vi "Consolidate Data Type.vi"(11 "Type in":T1) -> (3 "Type out":T1)   [LabVIEW 2020, in "hse-config.lvlib" / "config-base.lvclass"]
doc: "____\nHAMPEL SOFTWARE ENGINEERING v3.8.0 (2023-12-18 14:41)"
uses:
  config-base.lvclass
  <vilib>/Utility/Data Type/Type Definitions/Data Type.ctl
  config-base.lvclass/config-base.ctl
  <vilib>/Utility/Data Type/NI_Data Type.lvlib
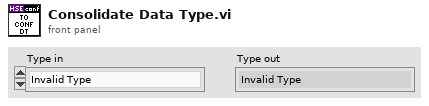
[diagram p1: front panel]
types:
  T1 = typedef "NI_Data Type.lvlib/Data Type.ctl" = enum8{"Invalid Type", "Void", "I8", "I16", "I32", "I64", "U8", "U16", "U32", "U64", "Single Float", "Double Float", "Extended Float", "Single Complex", "Double Complex", "Extended Complex", "Enum U8", "Enum U16", "Enum U32", "Enum U64", "Single Float With Unit", "Double Float With Unit", "Extended Float With Unit", "Single Complex with Unit", "Double Complex with Unit", "Extended Complex with Unit", "Boolean", "String", "Path", "Picture", "Tag", "Array", "Cluster", "Variant", "LV Variant", "Waveform", "Timestamp", "Digital Waveform", "Digital Data", "ExpressData", "Refnum", "External Data", "VI", "Poly VI", "LabVIEW Class Instance", "Fixed Point", "Set Collection", "Map Collection"}
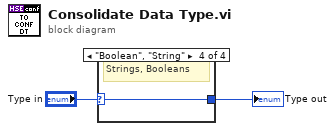
[diagram p0: block diagram]
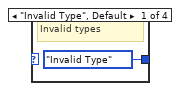
[diagram p2: hidden frame]
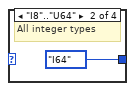
[diagram p3: hidden frame]
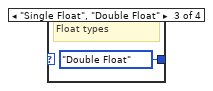
[diagram p4: hidden frame]
diagram:
  n1 = case shown="\"Boolean\", \"String\"" "Type in" {
    selector: "Type in" -> [_ _ _ w6]
    tunnel: [Data_Type."Invalid Type" ("Type") Data_Type."I64" ("Type") Data_Type."Double Float" ("Type") w6] -> w2
    frame "Invalid Type", Default {
      # "Invalid types"
    }
    frame "I8".."U64" {
      # "All integer types"
    }
    frame "Single Float", "Double Float" {
      # "Float types"
    }
    frame "Boolean", "String" {
      # "Strings, Booleans"
    }
  }
  "Type out" <- w2
